vi "Write configuration.vi"(8 "error in (no error)":errorcluster, 11 "AOTF in":refnum<class "AOTF.lvclass">) -> (0 "error out":errorcluster, 3 "AOTF out":refnum<class "AOTF.lvclass">)   [LabVIEW 2012, in "AOTF.lvclass"]
doc: "Writes the configuration cluster into the configuration file. Configuration file is XML-based. It's name is <component ID>.xml"
uses:
  AOTF.lvclass
  <vilib>/Distrio/Murmex/Murmex/Murmex.lvclass
  AOTF.lvclass/AOTF.ctl
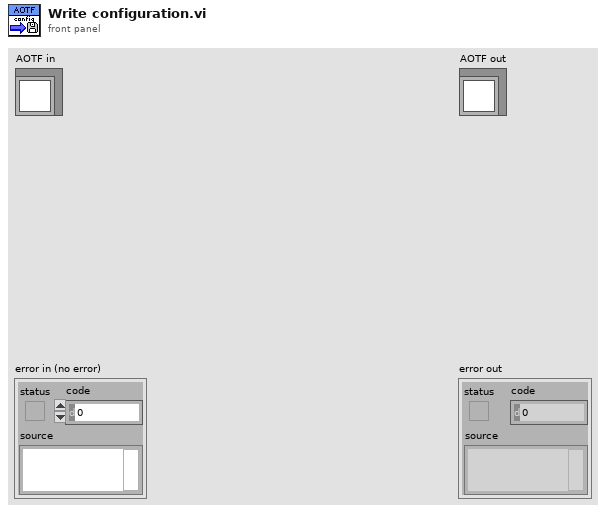
[diagram p1: front panel]
types:
  T1 = typedef "AOTF.lvclass/Configuration cluster.ctl" = cluster{"AO channel":tag, "DO lines":tag, "LUT path Cluster":cluster{"LUT path Array":path[]}}
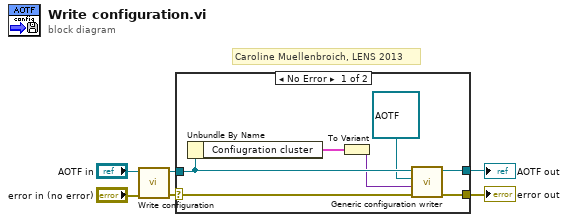
[diagram p0: block diagram]
diagram:
  # "Caroline Muellenbroich, LENS 2013"
  n1 = call-parent "Write configuration.vi"("error in (no error)"="error in (no error)", "Murmex in"="AOTF in") -> ("error out"=w4:errorcluster, "Murmex out"=w3:refnum<class "AOTF.lvclass">)  [unwired: 8 in]
  n2 = case shown="No Error" w4 {
    selector: w4 -> [w11 w14]
    tunnel: [w12 w15] -> w2
    tunnel: w3 -> [w10 w15]
    tunnel: [w13 w14] -> w1
    frame No Error {
      n3 = Unbundle By Name(w10) -> ("Confiugration cluster"=w9:T1)
      n4 = To Variant(anything=w9) -> (Variant=w8:variant)
      n5 = call <vilib>:"Generic configuration writer.vi"("error in (no error)"=w11, "configuration"=w8, "inheritance level"=refnum<class "AOTF.lvclass"> refnum ("AOTF"), "MurmexBase in"=w10) -> ("error out"=w13:errorcluster, "MurmexBase out"=w12:refnum<class "AOTF.lvclass">)  [unwired: 6 in]
    }
    frame Error {
    }
  }
  "error out" <- w1
  "AOTF out" <- w2
